vi "Write WindowFunction.vi"(8 "error in (no error)":errorcluster, 10 "window":T1 items=["Rectangle"=0, "Hanning"=1, "Hamming"=2, "Blackman-Harris"=3, "Exact Blackman"=4, "Blackman"=5, "Flat Top"=6, "4 Term B-Harris "=7, "7 Term B-Harris"=8, "Low Sidelobe"=9, "Blackman Nuttall"=11, "Triangle"=30, "Bartlett-Hanning"=31, "Bohman"=32, "Parzen"=33, "Welch"=34, "Kaiser"=60, "Dolph-Chebyshev"=61, "Gaussian"=62], 11 "FFT in":refnum<class "FFT.lvclass">) -> (0 "error out":errorcluster, 3 "FFT out":refnum<class "FFT.lvclass">)   [LabVIEW 2014, in "AnalysisPlugins.lvlib" / "FFT.lvclass"]
uses:
  FFT.lvclass
  <vilib>/Analysis/4window.llb/windowTd.ctl
  FFT.lvclass/FFT.ctl
  <vilib>/Analysis/NI_AALPro.lvlib
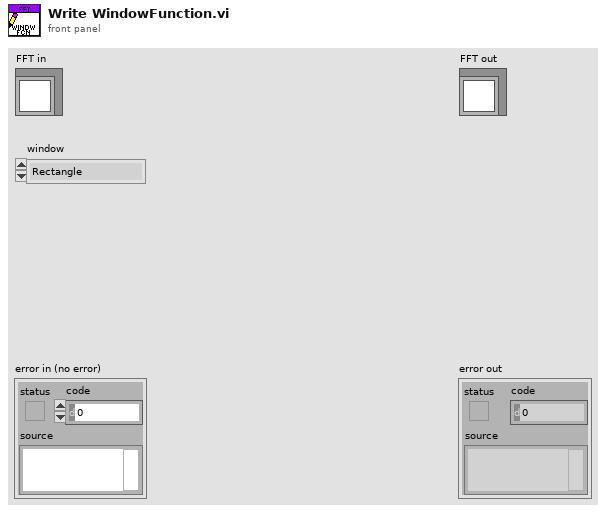
[diagram p1: front panel]
types:
  T1 = typedef "NI_AALPro.lvlib/windowTd.ctl" = u32
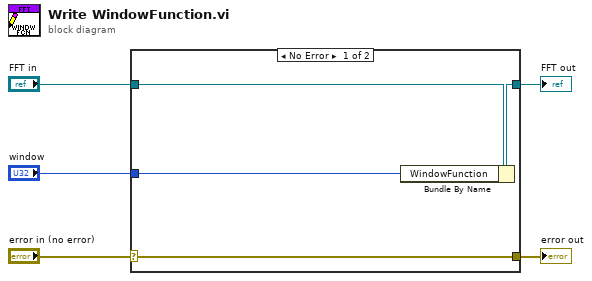
[diagram p0: block diagram]
diagram:
  n1 = case shown="No Error" "error in (no error)" {
    selector: "error in (no error)" -> [w9 w10]
    tunnel: [w9 w10] -> w4
    tunnel: [w7 w11] -> w2
    tunnel: "FFT in" -> [w8 w11]
    tunnel: "window" -> [w6 _]
    frame No Error {
      n2 = Bundle By Name(cluster=w8, "WindowFunction"=w6) -> (w7:refnum<class "FFT.lvclass">)
    }
    frame Error {
    }
  }
  "error out" <- w4
  "FFT out" <- w2
